vi "Raster_plot_v001.vi"() -> ()   [LabVIEW 2019]
panel:
  out "Raster plot":dbl(graph)
  out "Numeric received":dbl
  out "Message received":string
  in  "stop":bool
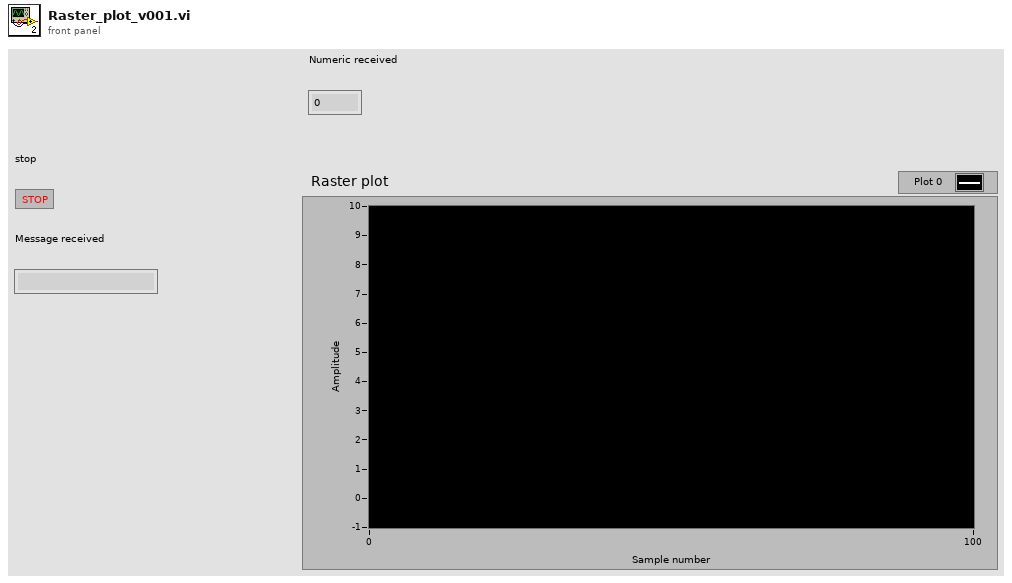
[diagram p1: front panel]
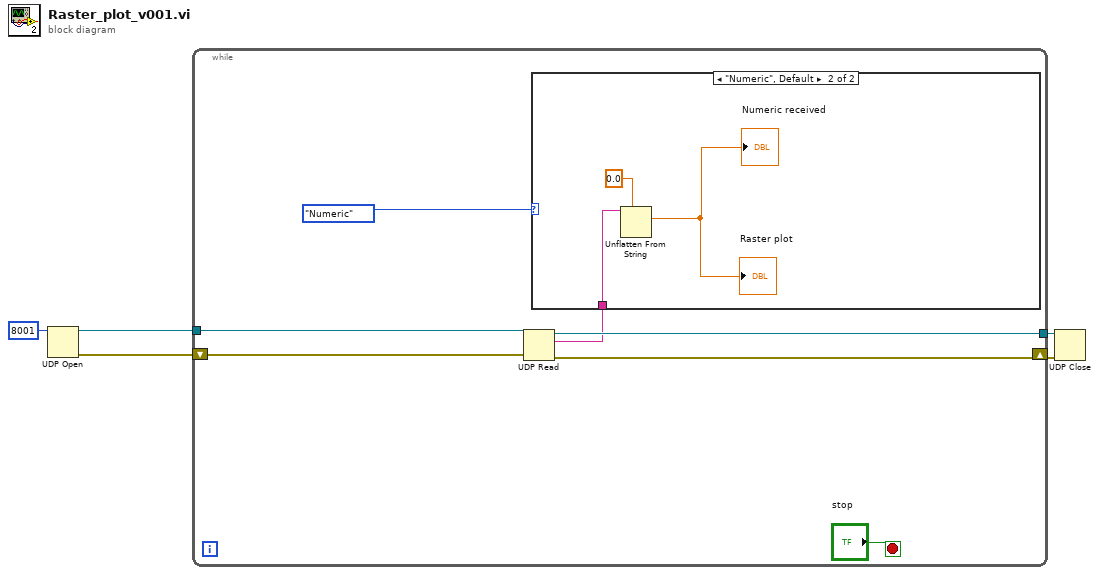
[diagram p0: block diagram]
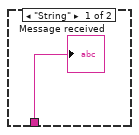
[diagram p2: hidden frame]
diagram:
  n1 = UDP Open(11:u16 8001 ("port")) -> (port=w3:refnum<k16>, 0:w5:errorcluster)  [unwired: 4 in, 1 out]
  n2 = while {
    shift-right: [w10] -> w4
    shift-left: w5 -> [w11]
    tunnel: w3 -> [w9]
    tunnel: [w8] -> w2
    stop <- "stop" stop-if-true
    n3 = UDP Read(connection ID=w9, 8:w11) -> (data out=w7:string, error out=w10:errorcluster, 3:w8:refnum<k16>)  [unwired: 2 in, 2 out]
    n4 = case shown="\"Numeric\", Default" enum16{"String", "Numeric"}."Numeric" ("Data interpreter") {
      tunnel: w7 -> [w13 w16]
      frame "String" {
        "Message received" <- w13
      }
      frame "Numeric", Default {
        n5 = Unflatten From String(type=0.0, binary string=w16) -> (value=→"Numeric received" →"Raster plot":dbl)  [unwired: 3 in, 2 out]
      }
    }
  }
  n6 = UDP Close(connection ID=w2, 8:w4) -> ()  [unwired: 2 out]
